vi "Connect.vi"(8 "error in":errorcluster, 11 "SimELoad in":refnum<class "SimEload.lvclass">) -> (0 "error out":errorcluster, 3 "SimELoad out":refnum<class "SimEload.lvclass">)   [LabVIEW 2019, in "SimELoad.lvlib" / "SimEload.lvclass"]
uses:
  SimEload.lvclass
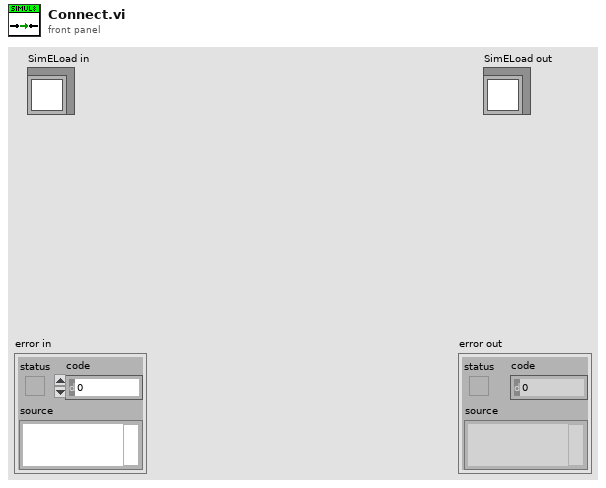
[diagram p1: front panel]
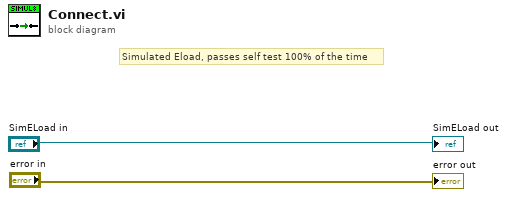
[diagram p0: block diagram]
diagram:
  # "Simulated Eload, passes self test 100% of the time"
  "error out" <- "error in"
  "SimELoad out" <- "SimELoad in"
